vi "FtpDirUploadSub.vi"(6 "パターン":string, 7 "アクティブ?(T)":bool=TRUE, 8 "error in (no error)":errorcluster caption="エラー入力（エラーなし）", 9 "ローカルディレクトリ":path, 10 "directory path":string caption="ディレクトリパス", 11 "ftp session":T1 caption="FTPセッション") -> (0 "error out":errorcluster caption="エラー出力", 3 "ftp session out":T1 caption="FTPセッション出力")   [LabVIEW 2014]
uses:
  <vilib>/FTP/NI_FTP.lvlib
  <vilib>/FTP/ftp0.llb/FTP Session.ctl
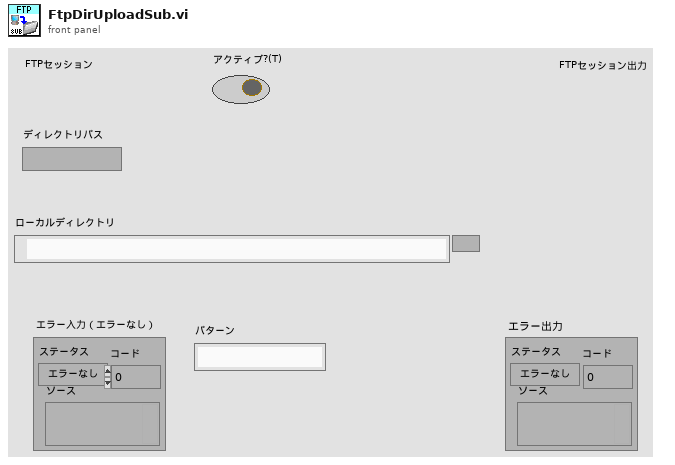
[diagram p1: front panel]
types:
  T1 = typedef "NI_FTP.lvlib/FTP Session.ctl" = refnum<k5>
  T2 = typedef "NI_FTP.lvlib/FTP File Info.ctl" = cluster{"type":enum16{"unknown", "file", "dir", "link"}, "permissions":string, "owner":string, "group":string, "size":i32, "date":string, "name":string, "link name":string}
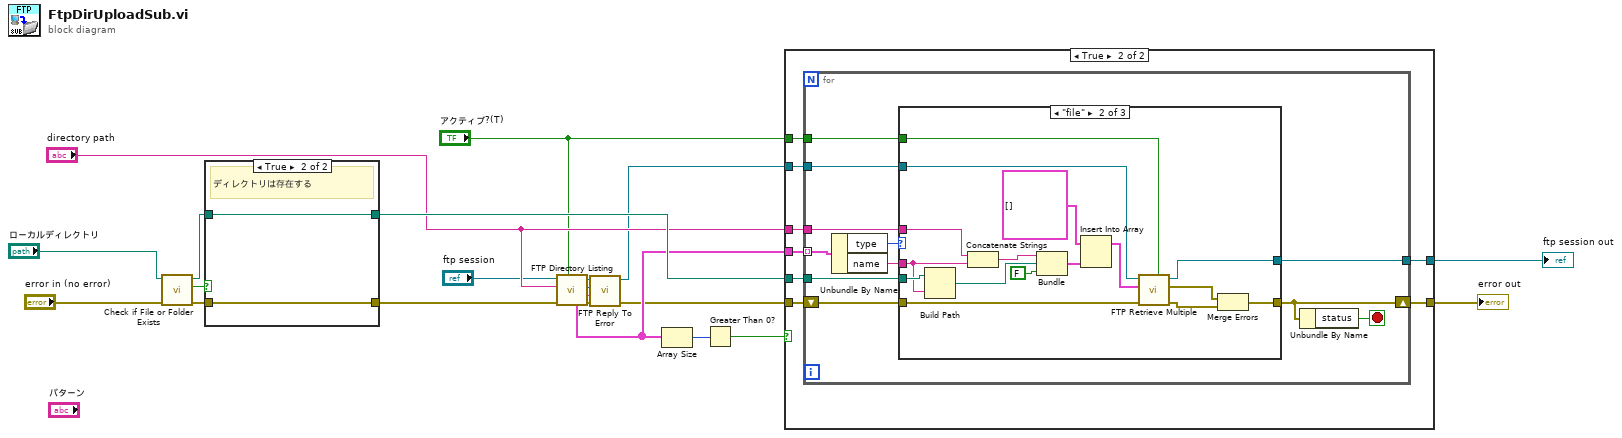
[diagram p0: block diagram]
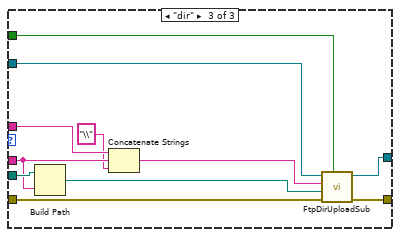
[diagram p4: hidden frame]
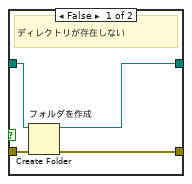
[diagram p5: hidden frame]
diagram:
  n1 = call <vilib>:"Check if File or Folder Exists.vi"("error in (no error)"="error in (no error)", "path"="ローカルディレクトリ") -> ("error out"=w13:errorcluster, "file or folder exists?"=w14:bool, "dup path"=w12:path)  [unwired: 7 in]
  n2 = case shown="TRUE" w14 {
    tunnel: w13 -> [w25 w27]
    tunnel: [w23 w27] -> w21
    tunnel: w12 -> [w24 w26]
    tunnel: [w22 w26] -> w18
    frame False {
      # "ディレクトリが存在しない"
      n3 = Create Folder "フォルダを作成"(path (use dialog)=w24, error in=w25) -> (created path=w22:path, error out=w23:errorcluster)  [unwired: 1 in, 1 out]
    }
    frame True {
      # "ディレクトリは存在する"
    }
  }
  n4 = call <vilib>:"FTP Directory Listing.vi"("active (T)"="アクティブ?(T)", "error in (no error)"=w21, "directory path"="directory path", "ftp session"="ftp session") -> ("error out"=w3:errorcluster, "reply string"=w4:string, "reply code"=w5:i32, "ftp session out"=w6:T1, "dir list"=w10:T2[])  [unwired: 3 in]
  n5 = call <vilib>:"FTP Reply To Error.vi"("error in (no error)"=w3, "reply string in"=w4, "reply code in"=w5, "ftp session"=w6) -> ("error out"=w1:errorcluster, "ftp session out"=w2:T1)  [unwired: 2 out]
  n6 = Array Size(array=w10) -> (size(s)=w9:i32)
  n7 = Greater Than 0?(x=w9) -> (x > 0?=w8:bool)
  n8 = case shown="TRUE" w8 {
    tunnel: "アクティブ?(T)" -> [_ w37]
    tunnel: w18 -> [_ w36]
    tunnel: [w29 w35] -> w15
    tunnel: w1 -> [w29 w34]
    tunnel: w2 -> [w28 w33]
    tunnel: [w28 w32] -> w17
    tunnel: "directory path" -> [_ w31]
    tunnel: w10 -> [_ w30]
    frame False {
    }
    frame True {
      n9 = for {
        tunnel: w30 -> [w40] mode=indexing
        tunnel: w31 -> [w46]
        tunnel: w37 -> [w45]
        tunnel: w36 -> [w44]
        shift-right: [w38] -> w35
        shift-left: w34 -> [w42]
        tunnel: w33 -> [w41]
        tunnel: [w39] -> w32
        stop <- w43 stop-if-true
        n10 = Unbundle By Name(w40) -> ("type"=w48:enum16{"unknown", "file", "dir", "link"}, "name"=w47:string)
        n11 = case shown="\"file\"" w48 {
          tunnel: w47 -> [_ w62 w71]
          tunnel: [w50 w54 w75] -> w38
          tunnel: w46 -> [_ w51 w77]
          tunnel: w45 -> [_ w55 w69]
          tunnel: w44 -> [_ w63 w72]
          tunnel: w42 -> [w50 w66 w74]
          tunnel: w41 -> [w49 w65 w68]
          tunnel: [w49 w56 w73] -> w39
          frame "unknown", Default {
          }
          frame "file" {
            n12 = Build Path(base path=w63, name or relative path=w62) -> (appended path=w61:path)
            n13 = Concatenate Strings(w51, w62) -> (w64:string)
            n14 = Bundle(w64, "appended path"=w61, FALSE) -> (w59:cluster{string, "appended path":path, bool})  [unwired: 1 in]
            n15 = Insert Into Array(array=cluster{string, "appended path":path, bool}[] [] ("配列"), new element=w59) -> (w58:cluster{string, "appended path":path, bool}[])  [unwired: 1 in]
            n16 = call <vilib>:"FTP Retrieve Multiple.vi"("active (T)"=w55, "error in (no error)"=w66, "file specifications"=w58, "ftp session"=w65) -> ("error out"=w53:errorcluster, "file errors"=w52:errorcluster[], "ftp session out"=w56:T1)  [unwired: 4 in, 1 out]
            n17 = Merge Errors(w52, w53) -> (w54:errorcluster)
          }
          frame "dir" {
            n18 = Build Path(base path=w72, name or relative path=w71) -> (appended path=w70:path)
            n19 = Concatenate Strings(w77, w71, "\\" ("文字列")) -> (w76:string)
            n20 = call "FtpDirUploadSub.vi"("アクティブ?(T)"=w69, "error in (no error)"=w74, "ローカルディレクトリ"=w70, "directory path"=w76, "ftp session"=w68) -> ("error out"=w75:errorcluster, "ftp session out"=w73:T1)  [unwired: 5 in]
          }
        }
        n21 = Unbundle By Name(w38) -> ("status"=w43:bool)
      }
    }
  }
  "error out" <- w15
  "ftp session out" <- w17
